vi "Kill All.vi"(4 "STOP":bool, 5 "VISA resource in":refnum<visa-resource-name>) -> (1 "STOP out":bool, 2 "VISA resource out":refnum<visa-resource-name>)   [LabVIEW 2012]
doc: "This is VI is configured to set all the heater outputs to OFF when STOP = True"
uses:
  Lake Shore 336.lvlib
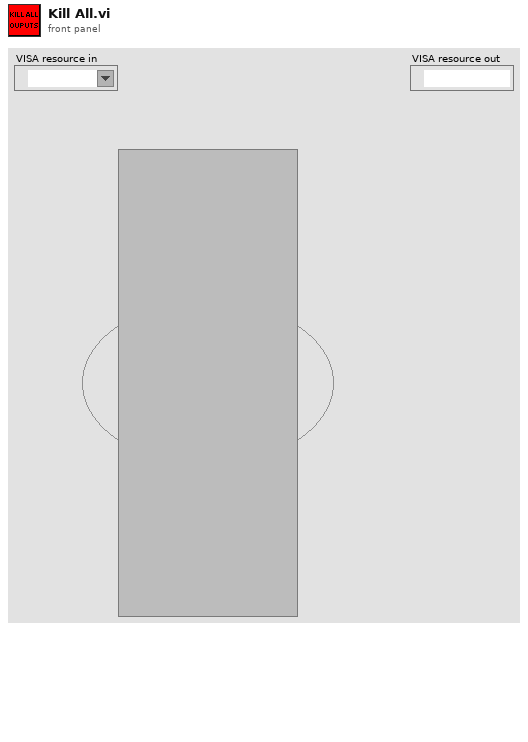
[diagram p1: front panel]
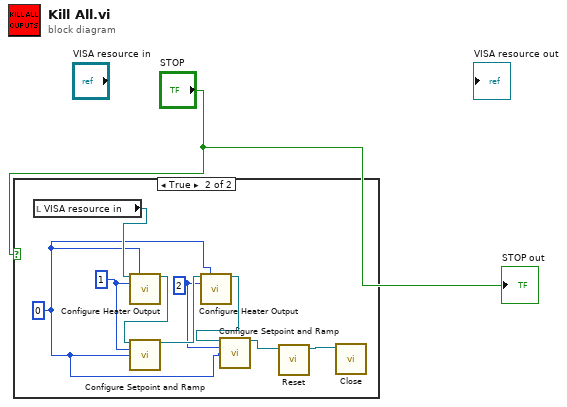
[diagram p0: block diagram]
diagram:
  n1 = case shown="True" "STOP" {
    frame False {
    }
    frame True {
      w5 = 2
      w8 = 1
      w4 = 0
      n2 = local read "VISA resource in"() -> (w10:refnum<visa-resource-name>)
      n3 = call "Configure Heater Output.vi"("VISA resource name"=w10, "Mode (0:Off)"=w4, "Heater Output (1:1)"=w8) -> ("VISA resource name out"=w9:refnum<visa-resource-name>)  [unwired: 11 in, 1 out]
      n4 = call "Configure Setpoint and Ramp.vi"("VISA resource name"=w9, "Output's Control Loop (1:1)"=w8, "Setpoint (0.00000)"=w4) -> ("VISA resource name out"=w7:refnum<visa-resource-name>)  [unwired: 11 in, 1 out]
      n5 = call "Configure Heater Output.vi"("VISA resource name"=w7, "Mode (0:Off)"=w4, "Heater Output (1:1)"=w5) -> ("VISA resource name out"=w6:refnum<visa-resource-name>)  [unwired: 11 in, 1 out]
      n6 = call "Configure Setpoint and Ramp.vi"("VISA resource name"=w6, "Output's Control Loop (1:1)"=w5, "Setpoint (0.00000)"=w4) -> ("VISA resource name out"=w3:refnum<visa-resource-name>)  [unwired: 11 in, 1 out]
      n7 = call "Reset.vi"("VISA resource name"=w3) -> ("VISA resource name out"=w2:refnum<visa-resource-name>)  [unwired: 9 in, 1 out]
      n8 = call "Close.vi"("VISA resource name"=w2) -> ()  [unwired: 10 in, 1 out]
    }
  }
  "STOP out" <- "STOP"
